vi "Write headers.vi"(8 "error in (no error)":errorcluster, 10 "headers":string, 11 "httpResponse in":refnum<class "httpResponse.lvclass">) -> (0 "error out":errorcluster, 3 "httpResponse out":refnum<class "httpResponse.lvclass">)   [LabVIEW 2020, in "httpClient.lvlib" / "httpResponse.lvclass"]
uses:
  httpResponse.lvclass
  httpResponse.lvclass/httpResponse.ctl
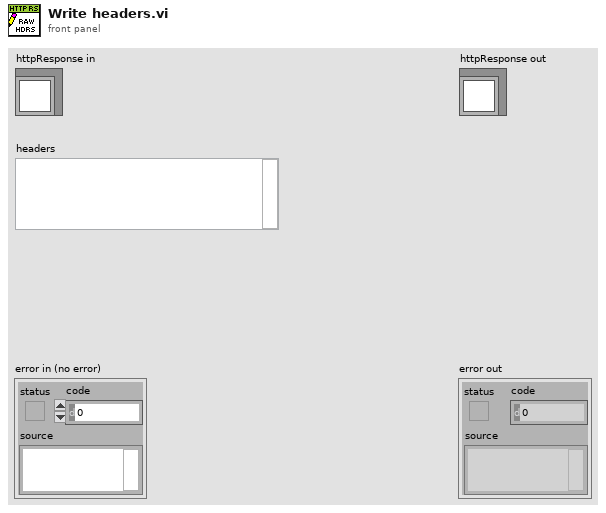
[diagram p1: front panel]
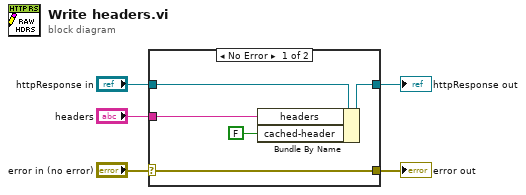
[diagram p0: block diagram]
diagram:
  n1 = case shown="No Error" "error in (no error)" {
    selector: "error in (no error)" -> [w10 w11]
    tunnel: [w10 w11] -> w4
    tunnel: [w6 w12] -> w2
    tunnel: "httpResponse in" -> [w9 w12]
    tunnel: "headers" -> [w8 _]
    frame No Error {
      n2 = Bundle By Name(cluster=w9, "headers"=w8, "cached-header"=FALSE ("cached")) -> (w6:refnum<class "httpResponse.lvclass">)
    }
    frame Error {
    }
  }
  "error out" <- w4
  "httpResponse out" <- w2
